vi "Ctor.vi"(8 "error in (no error)":errorcluster, 11 "StokePlotHandle in":refnum<class "BjusticePlotHandle.lvclass">) -> (0 "error out":errorcluster, 3 "StokePlotHandle out":refnum<class "BjusticePlotHandle.lvclass">)   [LabVIEW 2021, in "BjusticePlotHandle.lvclass"]
uses:
  BjusticePlotHandle.lvclass
  BjusticePlotHandle.lvclass/BjusticePlotHandle.ctl
  RocketPlotHandle/RocketPlotHandle.lvclass
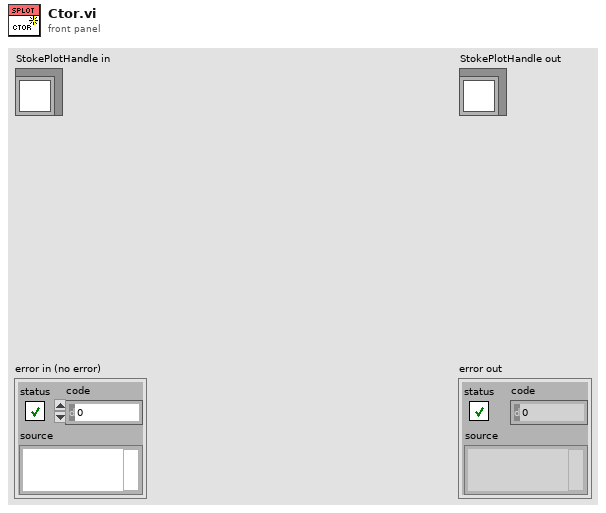
[diagram p1: front panel]
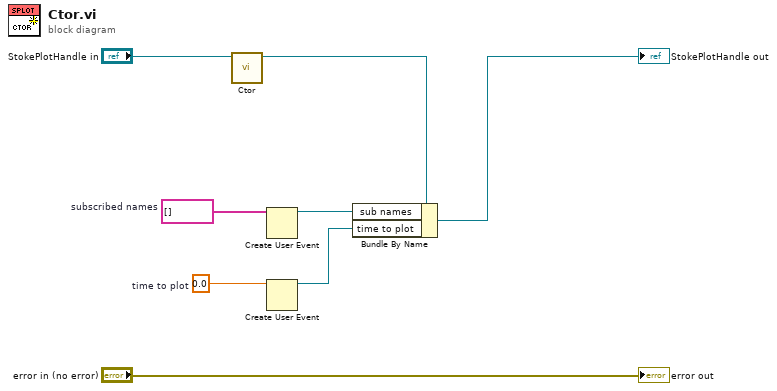
[diagram p0: block diagram]
diagram:
  w3 = 0.0  # time to plot
  w4 = string[] []  # subscribed names
  n1 = call-parent "Ctor.vi"("BluePlotHandle in"="StokePlotHandle in") -> ("BluePlotHandle out"=w5:refnum<class "BjusticePlotHandle.lvclass">)  [unwired: 9 in, 1 out]
  n2 = Create User Event(user event datatype=w4) -> (user event=w2:refnum<user-event>)  [unwired: 1 in, 1 out]
  n3 = Create User Event(user event datatype=w3) -> (user event=w1:refnum<user-event>)  [unwired: 1 in, 1 out]
  n4 = Bundle By Name(cluster=w5, "sub names"=w2, "time to plot"=w1) -> (→"StokePlotHandle out":refnum<class "BjusticePlotHandle.lvclass">)
  "error out" <- "error in (no error)"
